vi "test_Timer.vi"() -> ()   [LabVIEW 2009]
uses:
  modules/timer/car_Timer_Command_enum.ctl
panel:
  in  "Pause":bool
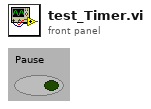
[diagram p1: front panel]
types:
  T1 = typedef "car_Timer_Command_enum.ctl" = enum16{"Start Timer", "Check Timer"}
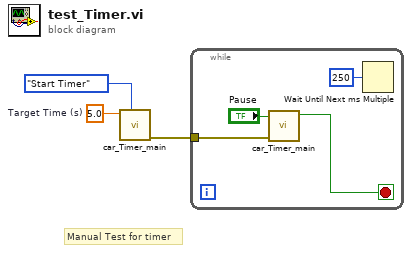
[diagram p0: block diagram]
diagram:
  w1 = 5.0  # Target Time (s)
  # "Manual Test for timer"
  n1 = call "car_Timer_main.vi"("Command (Check Timer)"=car_Timer_Command_enum."Start Timer", "Target Time (s)"=w1) -> ("error out"=w2:errorcluster)  [unwired: 8 in, 1 out]
  n2 = while {
    tunnel: w2 -> [w7]
    stop <- w5 stop-if-true
    n3 = call "car_Timer_main.vi"("error in (no error)"=w7, "Pause"="Pause") -> ("Elapsed"=w5:bool)  [unwired: 8 in, 1 out]
    n4 = Wait Until Next ms Multiple(millisecond multiple=u32 250) -> ()  [unwired: 1 out]
  }
